vi "ZAlign_MoveSelected.vi"(8 "error in (no error)":errorcluster, 10 "CtrlRefs":refnum<vi>[](array[refnum]) caption="Objects", 11 "Controls":refnum<vi>[](array[refnum]) caption="Objects") -> (0 "error out":errorcluster)   [LabVIEW 2014, in "ZAlign.lvlib"]
doc: "ZAlign.lvlib:ZAlign_GroupAndMovetoBack.vi\n----------------------------------------------\nDecos group an move to Back\n\nInputs:\n---------------------\n- error in (no error) : Cluster; \n- Objects : 1DArrayOfRefnum; \n- Panel : Refnum; \n\nOutputs:\n---------------------\n- error out : Cluster; \n\n----------------------------------------------\n16/03/2015\nZühlke Engineering AG\nCH-8952 Schlieren\nwww.zuehlke.com"
uses:
  ZAlign.lvlib
  <vilib>/Utility/miscctls.llb/LVPositionTypeDef.ctl
panel:
  # "Connector Pane"
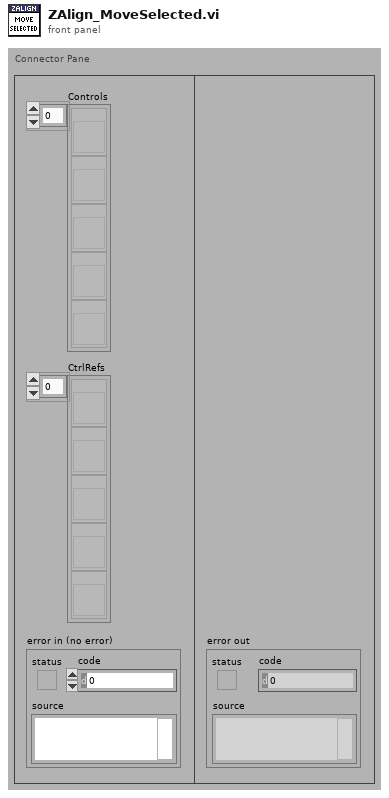
[diagram p1: front panel]
types:
  T1 = typedef "LVPositionTypeDef.ctl" = cluster{"Left":i32, "Top":i32}
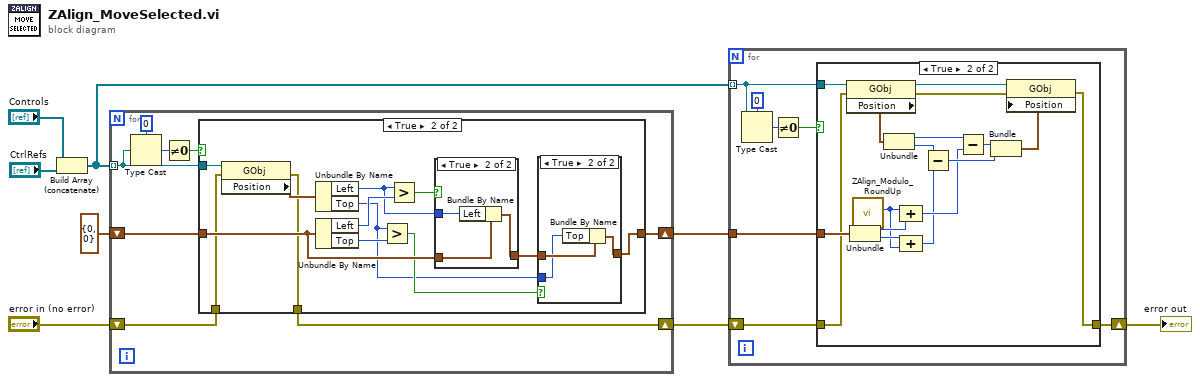
[diagram p0: block diagram]
diagram:
  n1 = Build Array (concatenate)("Controls", "CtrlRefs") -> (w1:refnum<vi>[])
  n2 = for {
    tunnel: w1 -> [w11] mode=indexing
    shift-right: [w15] -> w6
    shift-left: T1 {"Left"=0, "Top"=0} ("Position") -> [w16]
    shift-right: [w13] -> w5
    shift-left: "error in (no error)" -> [w14]
    n3 = Type Cast(type=0, x=w11) -> (*(type *) &x=w10:i32)
    n4 = Not Equal To 0?(x=w10) -> (x != 0?=w12:bool)
    n5 = case shown="True" w12 {
      tunnel: w16 -> [w18 w29]
      tunnel: [w18 w22] -> w15
      tunnel: w14 -> [w17 w21]
      tunnel: [w17 w20] -> w13
      tunnel: w11 -> [_ w19]
      frame False {
      }
      frame True {
        n6 = property class="GObj"(reference=w19, error in=w21) -> (error out=w20:errorcluster, "Position"=w31:T1)  [unwired: 1 out]
        n7 = Unbundle By Name(w31) -> ("Left"=w27:i32, "Top"=w23:i32)
        n8 = Unbundle By Name(w29) -> ("Left"=w30:i32, "Top"=w26:i32)
        n9 = Greater?(x=w23, y=w26) -> (0:w24:bool)
        n10 = Greater?(x=w27, y=w30) -> (0:w28:bool)
        n11 = case shown="True" w28 {
          tunnel: w29 -> [w36 w39]
          tunnel: [w36 w38] -> w25
          tunnel: w27 -> [_ w37]
          frame False {
          }
          frame True {
            n12 = Bundle By Name(cluster=w39, "Left"=w37) -> (w38:T1)
          }
        }
        n13 = case shown="True" w24 {
          tunnel: w25 -> [w32 w35]
          tunnel: [w32 w34] -> w22
          tunnel: w23 -> [_ w33]
          frame False {
          }
          frame True {
            n14 = Bundle By Name(cluster=w35, "Top"=w33) -> (w34:T1)
          }
        }
      }
    }
  }
  n15 = for {
    tunnel: w1 -> [w42] mode=indexing
    tunnel: w6 -> [w46]
    shift-right: [w44] -> w4
    shift-left: w5 -> [w45]
    n16 = Type Cast(type=0, x=w42) -> (*(type *) &x=w41:i32)
    n17 = Not Equal To 0?(x=w41) -> (x != 0?=w40:bool)
    n18 = case shown="True" w40 {
      tunnel: w46 -> [_ w62]
      tunnel: w45 -> [w47 w56]
      tunnel: [w47 w54] -> w44
      tunnel: w42 -> [_ w53]
      frame False {
      }
      frame True {
        n19 = property class="GObj"(reference=w53, error in=w56) -> (reference out=w60:refnum<vi>, error out=w55:errorcluster, "Position"=w64:T1)
        n20 = Unbundle(w62) -> ("Left"=w52:i32, "Top"=w50:i32)
        n21 = call "ZAlign_Modulo_RoundUp.vi"() -> ("Grid_Size"=w48:i32)  [unwired: 10 in, 1 out]
        n22 = Unbundle(w64) -> ("Left"=w61:i32, "Top"=w63:i32)
        n23 = Compound Arithmetic op=ADD(w48, w52) -> (w51:i32)
        n24 = Compound Arithmetic op=ADD(w50, w48) -> (w49:i32)
        n25 = Subtract(x=w63, y=w49) -> (x-y=w58:i32)
        n26 = Subtract(x=w61, y=w51) -> (x-y=w59:i32)
        n27 = Bundle(w59, w58) -> (w57:cluster{i32, i32})  [unwired: 1 in]
        n28 = property class="GObj"(reference=w60, error in=w55, "Position"=w57) -> (error out=w54:errorcluster)  [unwired: 1 out]
      }
    }
  }
  "error out" <- w4
